vi "ROI entry-Init trig ctrls.vi"(8 "error in (no error)":errorcluster) -> (0 "error out":errorcluster)   [LabVIEW 2017]
uses:
  ROI Entry screen/Globals/gl_ROI Entry UI globals.vi
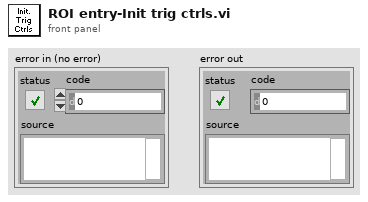
[diagram p1: front panel]
types:
  T1 = enum8{"Enabled", "Disabled", "Disabled and Grayed Out"}
  T2 = typedef "ROI entry screen ctrl refs cluster.ctl" = cluster{"Done button":refnum<vi>, "Imaging button":refnum<vi>, "Acquisition button":refnum<vi>, "POI dwell time (us)":refnum<vi>, "Scan dwell time per pixel (us)":refnum<vi>, "# of planes":refnum<vi>, "Zoom Ctrl":refnum<vi>, "Equal size":refnum<vi>, "Channel":refnum<vi>, "Image Display":refnum<vi>, "Z-Plane Selector":refnum<vi>, "Number of lines left":refnum<vi>, "Z-stack folder path":refnum<vi>, "POI Density":refnum<vi>, "Arb Plane Entry":refnum<vi>, "Whole plane":refnum<vi>, "Clear Last":refnum<vi>, "Clear All":refnum<vi>, "Trial Length (sec)":refnum<vi>, "Palette Type":refnum<vi>, "Intensity slider":refnum<vi>, "# POI":refnum<vi>, "Max Z Proj":refnum<vi>, "Zplane ind":refnum<vi>, "Wavelength (nm)":refnum<vi>, "Number of Trials":refnum<vi>, "Funct stim.trig.enable":refnum<vi>, "Funct stim.trig.delay (s)":refnum<vi>, "Line Mode":refnum<vi>, "Step size (µm)":refnum<vi>, "ROI move mode":refnum<vi>, "Cool-down time (s)":refnum<vi>, "Enable cool-down time":refnum<vi>, "Motor Z ind. (um)":refnum<vi>, "AOL Z ind. (um)":refnum<vi>, "Load Reference Image":refnum<vi>}
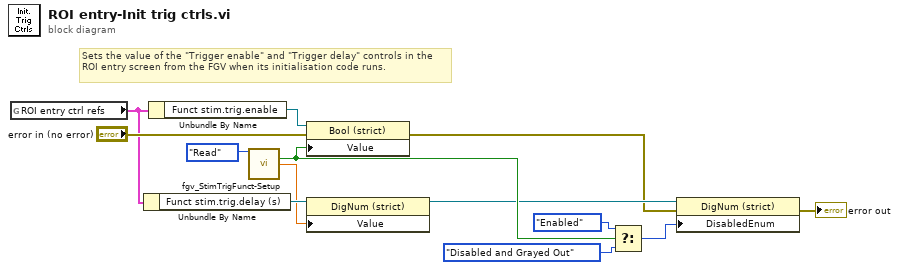
[diagram p0: block diagram]
diagram:
  # "Sets the value of the \"Trigger enable\" and \"Trigger delay\" controls in the ROI entry screen from the FGV when its initialisation code runs."
  n1 = global read "gl_ROI Entry UI globals.vi" "ROI entry ctrl refs"() -> (w10:T2)
  n2 = Unbundle By Name(w10) -> ("Funct stim.trig.delay (s)"=w11:refnum<vi>)
  n3 = Unbundle By Name(w10) -> ("Funct stim.trig.enable"=w9:refnum<vi>)
  n4 = call "fgv_StimTrigFunct-Setup.vi"("Function"=enum16{"Intialize", "Write", "Read", "Clear"}."Read") -> ("Live stim.trig.enable"=w6:bool, "Funct stim.trig.delay (sec)"=w1:dbl)  [unwired: 11 in, 2 out]
  n5 = property on="Property Node" class="Bool (strict)"(reference=w9, error in="error in (no error)", "Value"=w6) -> (error out=w3:errorcluster)  [unwired: 1 out]
  n6 = property on="Property Node" class="DigNum (strict)"(reference=w11, "Value"=w1) -> (reference out=w4:refnum<vi>)  [unwired: 1 in, 1 out]
  n7 = Select(t=T1."Enabled" ("Disabled"), s=w6, f=T1."Disabled and Grayed Out" ("Disabled")) -> (s? t:f=w8:T1)
  n8 = property on="Property Node" class="DigNum (strict)"(reference=w4, error in=w3, "DisabledEnum"=w8) -> (error out=→"error out":errorcluster)  [unwired: 1 out]
